vi "Main.vi"() -> ()   [LabVIEW 2018]
doc: "The myRIO Project template acquires acceleration data from the onboard accelerometer and displays the changes of acceleration values in a waveform chart."
uses:
  <vilib>/myRIO/Common/Instrument Driver Framework/myRIO v1.0/UART/vis/myRIO v1.0 Close UART.vi
  <vilib>/Utility/error.llb/Error Cluster From Error Code.vi
  <vilib>/myRIO/Common/Instrument Driver Framework/myRIO v1.0/PWM/vis/myRIO v1.0 Write PWM.vi
  <vilib>/myRIO/Common/Instrument Driver Framework/myRIO v1.0/DIO/vis/myRIO v1.0 Write DIO.vi
  <vilib>/myRIO/Common/Instrument Driver Framework/myRIO v1.0/AI/vis/myRIO v1.0 Read AI.vi
  <vilib>/myRIO/Common/Instrument Driver Framework/myRIO v1.0/DIO/vis/myRIO v1.0 Read DIO.vi
  <vilib>/myRIO/Common/Instrument Driver Framework/Utilities/vis/FPGA Ref Manager.vi
  <vilib>/myRIO/Common/Instrument Driver Framework/myRIO v1.0/myRIO v1.0 Reset FPGA.vi
  <vilib>/myRIO/Common/Instrument Driver Framework/myRIO v1.0/IRQ/vis/myRIO v1.0 IRQ Info FGV.vi
  <vilib>/myRIO/Common/Instrument Driver Framework/myRIO v1.0/IRQ/vis/myRIO v1.0 Timer IRQ Info FGV.vi
  <vilib>/myRIO/Common/Instrument Driver Framework/myRIO v1.0/IRQ/vis/myRIO v1.0 ISR Agent.vi
  <vilib>/myRIO/Instrument Drivers/Utilities/Utilities.lvlib
  <vilib>/myRIO/Instrument Drivers/Onboard IO/PWM/PWM.lvlib
  <vilib>/myRIO/Instrument Drivers/Onboard IO/AI/AI.lvlib
  <vilib>/myRIO/Instrument Drivers/Onboard IO/DIO/DIO.lvlib
panel:
  in  "ABORT STEPPER!!!!!":bool
  in  "Threshold Lower":dbl=2900.0
  in  "Threshold Upper":dbl=3200.0
  in  "Stepper frekvens":dbl=350.0
  out "ALL BOTTOM":bool
  out "ALL TOP":bool
  in  "Test bor (T = Amperestyring)":bool
  in  "DIR":bool
  in  "Endstops":bool
  in  "Manuel stepper?":bool
  in  "Enum":T1(ring)
  out "Batteri tilbage (%)":dbl
  out "Mean 200":dbl format="%0.2f"
  out "Duty Cycle":dbl
  in  "Styr manuelt?":bool=TRUE
  out "Waveform Chart":dbl(graph)
  out "Målt ampere":dbl
  in  "Bor - Frequency [Hz]":dbl=200.0
  in  "Bor - Duty Cycle":dbl=50.0
  out "error out":errorcluster
  in  "Stop":bool
  # "WIRING:\nBrun = GND\nOrange = PWM (A/DIO8)"
  # "STYRING AF SYSTEM!"
  # "100 = max\n50 = 0\n0 = -max"
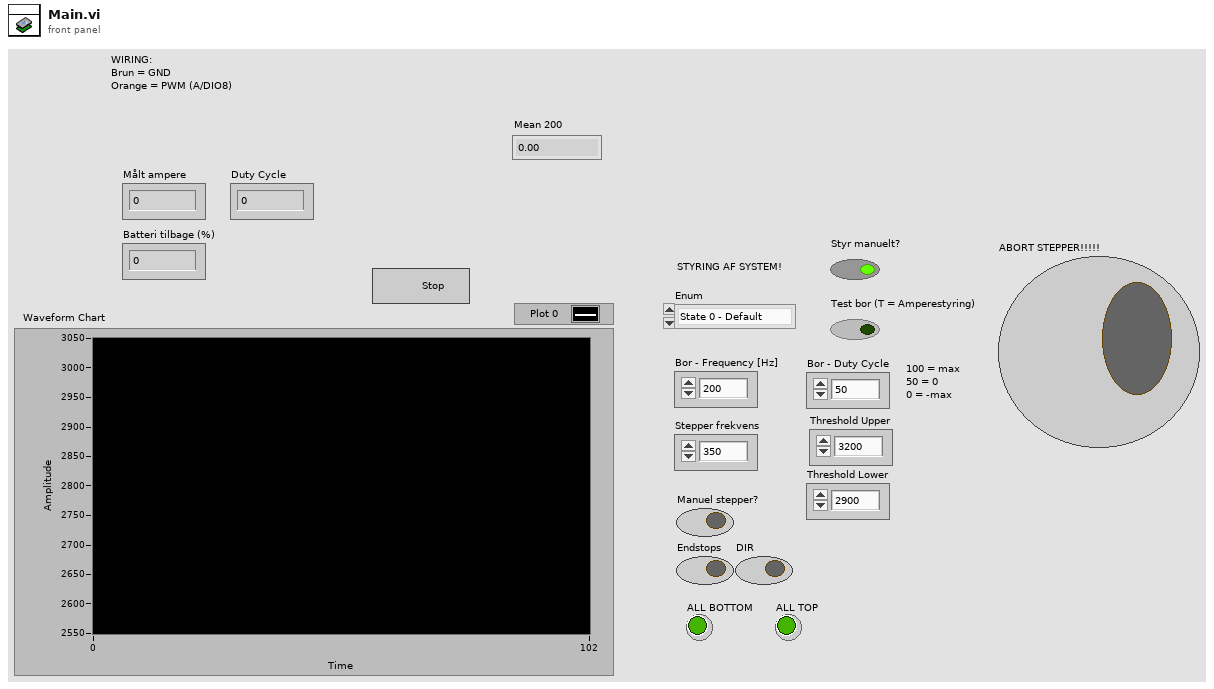
[diagram p1: front panel]
types:
  T1 = enum16{"State 0 - Default", "State 1 - Go down", "State 2 - Go up"}
  T2 = typedef "DIO.lvlib/DIO Reference.ctl" = cluster{"myRIO Reference":T3, "DIO Channels List":T7}
  T3 = typedef "myRIO Generic Hardware Reference.ctl" = cluster{"myRIO Model":T4, "myRIO Hardware Reference":T5}
  T4 = typedef "Hardware Version Enum.ctl" = enum16{"Unknown", "myRIO-1900", "myRIO-1950", "roboRIO", "NI ELVIS RIO CM", "ELVIS III"}
  T5 = typedef "myRIO v1.0 Reference.ctl" = cluster{"Generic FPGA Reference":T6, "Allow multiple opens":bool}
  T6 = typedef "Generic FPGA Reference.ctl" = refnum<k20>
  T7 = typedef "DIO Channels List.ctl" = T8[]
  T8 = typedef "DIO Channels Enum.ctl" = enum16{"Not Connected", "C/DIO0", "C/DIO1", "C/DIO2", "C/DIO3", "C/DIO4", "C/DIO5", "C/DIO6", "C/DIO7", "A/DIO0", "A/DIO1", "A/DIO2", "A/DIO3", "A/DIO4", "A/DIO5", "A/DIO6", "A/DIO7", "A/DIO8", "A/DIO9", "A/DIO10", "A/DIO11", "A/DIO12", "A/DIO13", "A/DIO14", "A/DIO15", "A/DIO16", "A/DIO17", "A/DIO18", "A/DIO19", "B/DIO0", "B/DIO1", "B/DIO2", "B/DIO3", "B/DIO4", "B/DIO5", "B/DIO6", "B/DIO7", "B/DIO8", "B/DIO9", "B/DIO10", "B/DIO11", "B/DIO12", "B/DIO13", "B/DIO14", "B/DIO15", "B/DIO16", "B/DIO17", "B/DIO18", "B/DIO19", "LED0", "LED1", "LED2", "LED3", "Button0", "DIO/DIO0", "DIO/DIO1", "DIO/DIO2", "DIO/DIO3", "DIO/DIO4", "DIO/DIO5", "DIO/DIO6", "DIO/DIO7", "DIO/DIO8", "DIO/DIO9", "SPI/CS0", "SPI/CS1", "SPI/CS2", "SPI/CS3", "LED RADIO (Green)", "LED RADIO (Red)", "LED COMM (Green)", "LED COMM (Red)", "LED MODE (Green)", "LED MODE (Red)"}
  T9 = typedef "PWM.lvlib/PWM Reference.ctl" = cluster{"myRIO Reference":T3, "PWM Channels Enum":T10, "PWM Configuration":T11}
  T10 = typedef "PWM Channels Enum.ctl" = enum16{"Not Connected", "C/PWM0", "C/PWM1", "A/PWM0", "A/PWM1", "A/PWM2", "A/PWM3", "A/PWM4", "A/PWM5", "A/PWM6", "A/PWM7", "A/PWM8", "A/PWM9", "A/PWM10", "A/PWM11", "A/PWM12", "A/PWM13", "A/PWM14", "A/PWM15", "A/PWM16", "A/PWM17", "A/PWM18", "A/PWM19", "B/PWM0", "B/PWM1", "B/PWM2", "B/PWM3", "B/PWM4", "B/PWM5", "B/PWM6", "B/PWM7", "B/PWM8", "B/PWM9", "B/PWM10", "B/PWM11", "B/PWM12", "B/PWM13", "B/PWM14", "B/PWM15", "B/PWM16", "B/PWM17", "B/PWM18", "B/PWM19", "PWM/PWM0", "PWM/PWM1", "PWM/PWM2", "PWM/PWM3", "PWM/PWM4", "PWM/PWM5", "PWM/PWM6", "PWM/PWM7", "PWM/PWM8", "PWM/PWM9"}
  T11 = typedef "PWM.lvlib/PWM Configuration.ctl" = cluster{"Frequency":dbl, "Duty Cycle":dbl}
  T12 = typedef "Accelerometer.lvlib/Accelerometer Reference.ctl" = cluster{"myRIO Reference":T3, "Accelerometer Channels List":T13, "LSB Weight":dbl}
  T13 = typedef "Accelerometer Channels List.ctl" = T14[]
  T14 = typedef "Accelerometer Channels Enum.ctl" = enum16{"Not Connected", "X-Axis", "Y-Axis", "Z-Axis"}
  T15 = typedef "AI.lvlib/AI Reference.ctl" = cluster{"myRIO Reference":T3, "AI Channels List":T16, "AI Scaling Constants List":T18}
  T16 = typedef "AI Channels List.ctl" = T17[]
  T17 = typedef "AI Channels Enum.ctl" = enum16{"Not Connected", "AudioIn/Left", "AudioIn/Right", "C/AI0", "C/AI1", "A/AI0", "A/AI1", "A/AI2", "A/AI3", "A/AI4", "A/AI5", "A/AI6", "A/AI7", "B/AI0", "B/AI1", "B/AI2", "B/AI3", "B/AI4", "B/AI5", "B/AI6", "B/AI7", "AI/AI0", "AI/AI1", "AI/AI2", "AI/AI3", "A/AI0 (DIFF)", "A/AI1 (DIFF)", "A/AI2 (DIFF)", "A/AI3 (DIFF)", "B/AI0 (DIFF)", "B/AI1 (DIFF)", "B/AI2 (DIFF)", "B/AI3 (DIFF)"}
  T18 = typedef "Analog Scaling Constants List.ctl" = T19[]
  T19 = typedef "Analog Scaling Constants.ctl" = cluster{"LSB Weight (Volts)":dbl, "Offset (Volts)":dbl, "Signed?":bool}
  T20 = typedef "SPI.lvlib/SPI Reference.ctl" = cluster{"myRIO Reference":T3, "SPI Channels Enum":T21, "SPI Configuration":T22}
  T21 = typedef "SPI Channels Enum.ctl" = enum16{"Not Connected", "A/SPI", "B/SPI", "SPI/SPI"}
  T22 = typedef "SPI.lvlib/SPI Configuration.ctl" = cluster{"Frequency [Hz]":dbl, "Clock Phase":T23, "Clock Polarity":T24, "Data Direction":T25, "Frame Length":T26}
  T23 = typedef "SPI Clock Phase.ctl" = enum8{"Leading", "Trailing"}
  T24 = typedef "SPI Clock Polarity.ctl" = enum8{"Low", "High"}
  T25 = typedef "SPI Data Direction.ctl" = enum8{"Most significant bit first", "Least significant bit first"}
  T26 = typedef "SPI Frame Length.ctl" = u8
  T27 = cluster{"B/DIO0 - Stepper Direction":T2, "B/DIO1 - Stepper1 Enable":T2, "B/DIO2 - Stepper2 Enable":T2, "B/DIO3 - Stepper3 Enable":T2, "B/DIO4 - Endstop Stepper1 Top":T2, "B/DIO11 - Endstop Stepper1 Bund":T2, "B/DIO12 - Endstop Stepper2 Top":T2, "B/DIO13 - Endstop Stepper2 Bund":T2, "B/DIO14 - Endstop Stepper3 Top":T2, "B/DIO15 - Endstop Stepper3 Bund":T2, "A/DIO0 - Cooler":T2, "A/DIO1 - Beacon drop (dio1)":T2, "A/DIO2 - Beacon drop (dio0)":T2, "A/DIO3 - QuickRelease (dio1)":T2, "A/DIO4 - QuickRelease (dio0)":T2, "A/DIO11 - LiDAR SPI CS":T2, "B/PWM0 - Stepper":T9, "B/PWM1 - Drill":T9, "A/PWM0 - Servo_Roll":T9, "A/PWM1 - Servo_Yaw":T9, "Acc. X-axis":T12, "Acc. Y-axis":T12, "B/AI0 - Drone Grounded F3":T15, "B/AI1 - Drone Drill Gear F4":T15, "B/AI2 - Beacon Drop F5":T15, "B/AI3 - Drone Drill Boost F6":T15, "A/AI0 - Drone Stepper F8":T15, "A/AI1 - Beacon Wiper":T15, "A/AI2 - QuickRelease Wiper":T15, "A/AI3 - Drill Current":T15, "A/SPI - LiDAR":T20, "B/UART - XBee":refnum<visa-resource-name>, "A/UART - A3 GPS":refnum<visa-resource-name>, "RIO Flashing LEDs":T2}
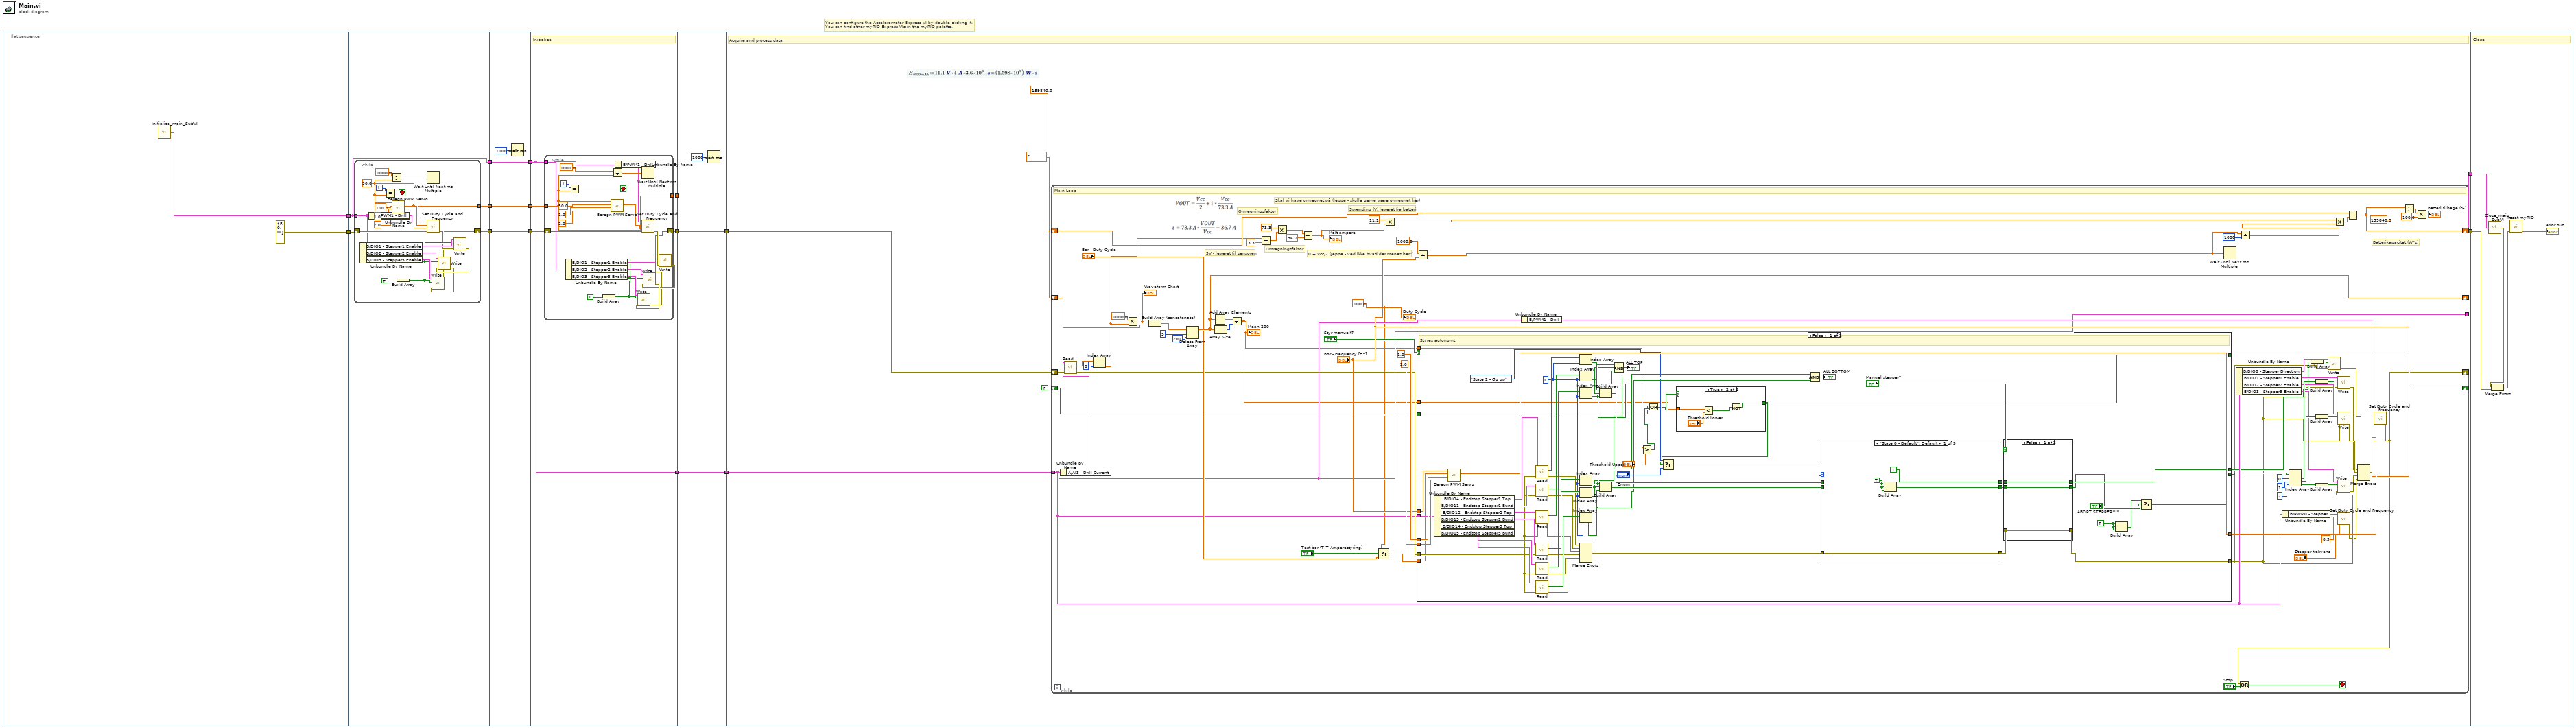
[diagram p0: block diagram]
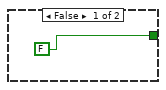
[diagram p2: hidden frame]
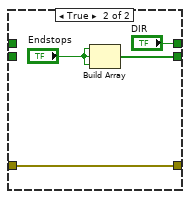
[diagram p3: hidden frame]
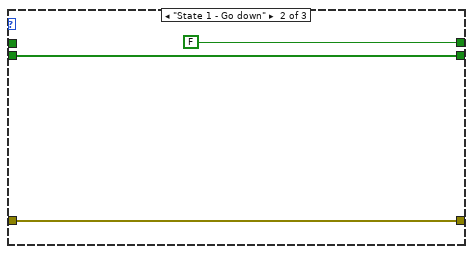
[diagram p4: hidden frame]
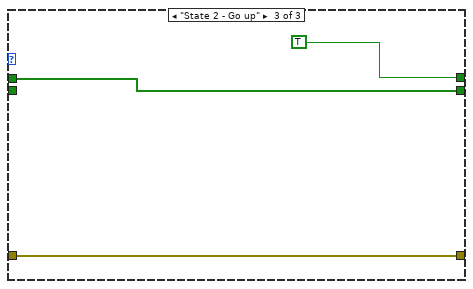
[diagram p5: hidden frame]
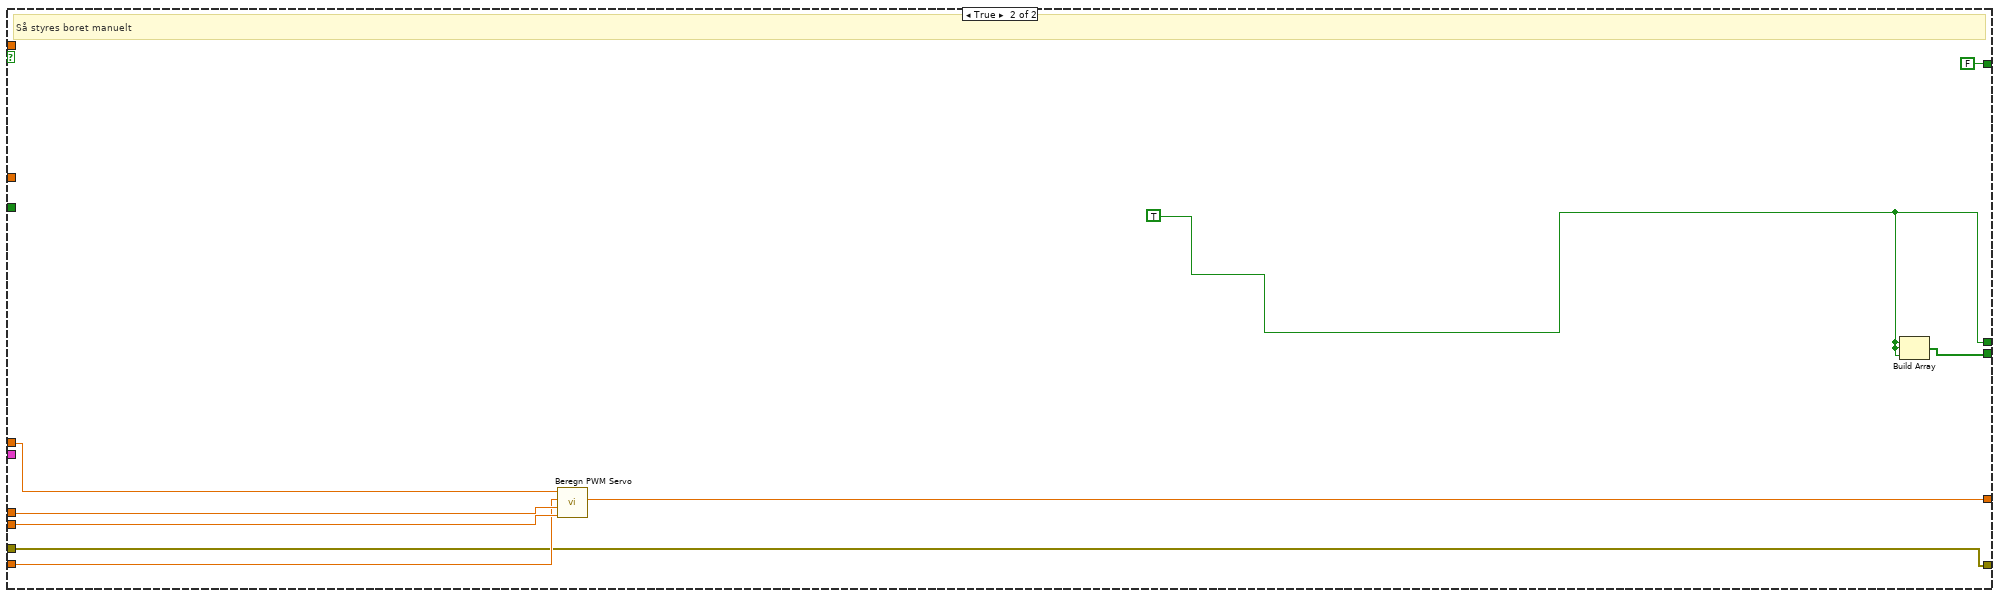
[diagram p6: hidden frame]
diagram:
  # "You can configure the Accelerometer Express VI by double-clicking it.\nYou can find other myRIO Express VIs in the myRIO palette."
  n1 = flat-sequence {
    tunnel: [w17] -> w8
    tunnel: [errorcluster {"status"=FALSE, "code"=0, "source"=""} ("error constant")] -> w2
    tunnel: [w21] -> w13
    tunnel: [w20] -> w11
    tunnel: w8 -> [w19]
    tunnel: [w19] -> w7
    tunnel: w2 -> [w18]
    tunnel: [w45] -> w14
    tunnel: w13 -> [w45]
    tunnel: [w44] -> w12
    tunnel: w11 -> [w44]
    tunnel: w7 -> [w43]
    tunnel: [w43] -> w6
    tunnel: w14 -> [w51]
    tunnel: w12 -> [w50]
    tunnel: [w48] -> w10
    tunnel: [w49] -> w9
    tunnel: w6 -> [w47]
    tunnel: [w47] -> w4
    tunnel: w10 -> [w73]
    tunnel: w9 -> [_]
    tunnel: [w74] -> w5
    tunnel: w4 -> [w74]
    tunnel: [w73] -> w3
    tunnel: [w82] -> w15
    tunnel: w5 -> [w79]
    tunnel: w3 -> [w78]
    tunnel: [w77] -> w1
    tunnel: w15 -> [w251]
    tunnel: w1 -> [w249]
    frame #0 {
      n2 = call "Initialize_main_SubVI.vi"() -> ("output cluster"=w17:T27)
    }
    frame #1 {
      n3 = while {
        tunnel: [w35] -> w21
        shift-right: [w22] -> w20
        shift-left: w18 -> [w38]
        tunnel: w19 -> [w31]
        i -> [w37]
        stop <- w33 stop-if-true
        w35 = 50.0 ("Frequency [Hz]")
        n4 = Unbundle By Name(w31) -> ("B/DIO1 - Stepper1 Enable"=w29:T2, "B/DIO2 - Stepper2 Enable"=w28:T2, "B/DIO3 - Stepper3 Enable"=w27:T2)
        n5 = Unbundle By Name(w31) -> ("B/PWM1 - Drill"=w32:T9)
        n6 = Equal?(x=w37, y=w35) -> (x = y?=w33:bool)
        n7 = Divide(x=1000.0, y=w35) -> (x/y=w36:dbl)
        n8 = call "Beregn PWM Servo.vi"("Max (ms puls bredde)"=2.0, "Min (ms puls bredde)"=1.0, "Duty Cycle"=100.0, "Frekvens"=w35) -> ("Output Dutycycle til PWM Servo"=w39:dbl)  [unwired: 7 in]
        n9 = Build Array(TRUE) -> (w26:bool[])
        n10 = Wait Until Next ms Multiple(millisecond multiple=w36) -> ()  [unwired: 1 out]
        n11 = call <vilib>:"Set Duty Cycle and Frequency.vi"("error in (no error)"=w38, "Frequency [Hz]"=w35, "Duty Cycle"=w39, "PWM Ref In"=w32) -> ("error out"=w25:errorcluster)  [unwired: 5 in, 1 out]
        n12 = call <vilib>:"Write.vi"("error in (no error)"=w25, "Values"=w26, "DIO Ref In"=w29) -> ("error out"=w24:errorcluster)  [unwired: 6 in, 1 out]
        n13 = call <vilib>:"Write.vi"("error in (no error)"=w24, "Values"=w26, "DIO Ref In"=w28) -> ("error out"=w23:errorcluster)  [unwired: 6 in, 1 out]
        n14 = call <vilib>:"Write.vi"("error in (no error)"=w23, "Values"=w26, "DIO Ref In"=w27) -> ("error out"=w22:errorcluster)  [unwired: 6 in, 1 out]
      }
    }
    frame #2 {
      n15 = Wait (ms)(milliseconds to wait=u32 1000) -> ()  [unwired: 1 out]
    }
    frame #3 {
      # "Initialize"
      n16 = while {
        tunnel: [w63] -> w49
        shift-right: [w54] -> w48
        shift-left: w50 -> [w68]
        tunnel: w51 -> [w63]
        tunnel: w47 -> [w56]
        i -> [w67]
        stop <- w64 stop-if-true
        n17 = Unbundle By Name(w56) -> ("B/DIO1 - Stepper1 Enable"=w53:T2, "B/DIO2 - Stepper2 Enable"=w58:T2, "B/DIO3 - Stepper3 Enable"=w59:T2)
        n18 = Equal?(x=w67, y=w63) -> (x = y?=w64:bool)
        n19 = Build Array(TRUE) -> (w52:bool[])
        n20 = call "Beregn PWM Servo.vi"("Max (ms puls bredde)"=2.0, "Min (ms puls bredde)"=1.0, "Duty Cycle"=50.0, "Frekvens"=w63) -> ("Output Dutycycle til PWM Servo"=w69:dbl)  [unwired: 7 in]
        n21 = Divide(x=1000.0, y=w63) -> (x/y=w66:dbl)
        n22 = Unbundle By Name(w56) -> ("B/PWM1 - Drill"=w62:T9)
        n23 = Wait Until Next ms Multiple(millisecond multiple=w66) -> ()  [unwired: 1 out]
        n24 = call <vilib>:"Set Duty Cycle and Frequency.vi"("error in (no error)"=w68, "Frequency [Hz]"=w63, "Duty Cycle"=w69, "PWM Ref In"=w62) -> ("error out"=w55:errorcluster)  [unwired: 5 in, 1 out]
        n25 = call <vilib>:"Write.vi"("error in (no error)"=w55, "Values"=w52, "DIO Ref In"=w53) -> ("error out"=w60:errorcluster)  [unwired: 6 in, 1 out]
        n26 = call <vilib>:"Write.vi"("error in (no error)"=w60, "Values"=w52, "DIO Ref In"=w58) -> ("error out"=w61:errorcluster)  [unwired: 6 in, 1 out]
        n27 = call <vilib>:"Write.vi"("error in (no error)"=w61, "Values"=w52, "DIO Ref In"=w59) -> ("error out"=w54:errorcluster)  [unwired: 6 in, 1 out]
      }
    }
    frame #4 {
      n28 = Wait (ms)(milliseconds to wait=u32 1000) -> ()  [unwired: 1 out]
    }
    frame #5 {
      # "Acquire and process data"
      n29 = while {
        shift-right: [w118] -> w82
        shift-left: w78 -> [w153]
        shift-right: [w143] -> _
        shift-left: dbl[] [] -> [w155]
        shift-right: [w128] -> _
        shift-left: 159840.0 -> [w129]
        tunnel: w79 -> [w115]
        tunnel: [w115] -> w77
        shift-right: [w86] -> _
        shift-left: FALSE ("t") -> [w85]
        stop <- w158 stop-if-true
        w83 = 100.0 ("upper limit")
        # "Batterikapacitet (W*s)"
        # "Spænding (V) leveret fra batteri"
        # "Omregningsfaktor"
        # "Omregningsfaktor"
        # "5V - leveret til sensoren"
        # "Skal vi have omregnet på (Jeppe - skulle gerne være omregnet her)"
        # "0 = Vcc/2 (Jeppe - ved ikke hvad der menes her?)"
        # "Main Loop"
        n30 = Unbundle By Name(w115) -> ("A/AI3 - Drill Current"=w121:T15)
        n31 = call <vilib>:"Read.vi"("error in (no error)"=w153, "AI Ref In"=w121) -> ("error out"=w119:errorcluster, "Values"=w152:dbl[])  [unwired: 7 in, 1 out]
        n32 = Index Array(array=w152, index=0) -> (element=w88:dbl)
        n33 = Multiply(x=1000.0, y=w88) -> (x*y=w141:dbl)
        "Waveform Chart" <- w141
        n34 = Build Array (concatenate)(w141, w155) -> (w146:dbl[])
        n35 = Delete From Array(array=w146, length=5, index=200) -> (array with subset deleted=w143:dbl[])  [unwired: 1 out]
        n36 = Add Array Elements(numeric array=w143) -> (sum=w145:dbl)
        n37 = Array Size(array=w143) -> (size(s)=w144:i32)
        n38 = Divide(x=w145, y=w144) -> (x/y=w84:dbl)
        "Mean 200" <- w84
        n39 = Divide(x=w88, y=3.3) -> (x/y=w139:dbl)
        n40 = Multiply(x=73.3, y=w139) -> (x*y=w137:dbl)
        n41 = Subtract(x=w137, y=36.7) -> (x-y=w134:dbl)
        "Målt ampere" <- w134
        n42 = Select(t=w83, s="Test bor (T = Amperestyring)", f="Bor - Duty Cycle") -> (s? t:f=w116:dbl)
        n43 = Multiply(x=11.1, y=w134) -> (x*y=w133:dbl)
        n44 = Divide(x=1000.0, y="Bor - Frequency [Hz]") -> (x/y=w87:dbl)
        n45 = case shown="False" "Styr manuelt?" {
          tunnel: 2.0 ("Max (ms puls bredde)") -> [w217 w248]
          tunnel: 1.0 ("Min (ms puls bredde)") -> [w215 w247]
          tunnel: [w214 w246] -> w151
          tunnel: "Bor - Frequency [Hz]" -> [w216 w245]
          tunnel: w115 -> [w195 _]
          tunnel: w119 -> [w194 w241]
          tunnel: w116 -> [w177 w244]
          tunnel: [w160 w242] -> w98
          tunnel: [w176 w241] -> w93
          tunnel: [w175 w243] -> w94
          tunnel: w84 -> [w171 _]
          tunnel: [w166 FALSE ("t")] -> w86
          tunnel: w85 -> [w169 _]
          tunnel: w84 -> [w167 _]
          frame False {
            w162 = TRUE
            w201 = 0 ("index")
            # "Styres autonomt"
            n46 = Unbundle By Name(w195) -> ("B/DIO4 - Endstop Stepper1 Top"=w213:T2, "B/DIO11 - Endstop Stepper1 Bund"=w212:T2, "B/DIO12 - Endstop Stepper2 Top"=w211:T2, "B/DIO13 - Endstop Stepper2 Bund"=w210:T2, "B/DIO14 - Endstop Stepper3 Top"=w209:T2, "B/DIO15 - Endstop Stepper3 Bund"=w208:T2)
            n47 = call "Beregn PWM Servo.vi"("Max (ms puls bredde)"=w217, "Min (ms puls bredde)"=w215, "Duty Cycle"=w177, "Frekvens"=w216) -> ("Output Dutycycle til PWM Servo"=w214:dbl)  [unwired: 7 in]
            n48 = call <vilib>:"Read.vi"("error in (no error)"=w194, "DIO Ref In"=w213) -> ("error out"=w193:errorcluster, "Values"=w202:bool[])  [unwired: 7 in, 1 out]
            n49 = call <vilib>:"Read.vi"("error in (no error)"=w194, "DIO Ref In"=w212) -> ("error out"=w192:errorcluster, "Values"=w203:bool[])  [unwired: 7 in, 1 out]
            n50 = call <vilib>:"Read.vi"("error in (no error)"=w194, "DIO Ref In"=w211) -> ("error out"=w191:errorcluster, "Values"=w204:bool[])  [unwired: 7 in, 1 out]
            n51 = call <vilib>:"Read.vi"("error in (no error)"=w194, "DIO Ref In"=w210) -> ("error out"=w190:errorcluster, "Values"=w205:bool[])  [unwired: 7 in, 1 out]
            n52 = call <vilib>:"Read.vi"("error in (no error)"=w194, "DIO Ref In"=w209) -> ("error out"=w189:errorcluster, "Values"=w206:bool[])  [unwired: 7 in, 1 out]
            n53 = call <vilib>:"Read.vi"("error in (no error)"=w194, "DIO Ref In"=w208) -> ("error out"=w188:errorcluster, "Values"=w207:bool[])  [unwired: 7 in, 1 out]
            n54 = Index Array(array=w202, index=w201) -> (element=w185:bool)
            n55 = Index Array(array=w204, index=w201) -> (element=w184:bool)
            n56 = Index Array(array=w206, index=w201) -> (element=w183:bool)
            n57 = Index Array(array=w203, index=w201) -> (element=w180:bool)
            n58 = Index Array(array=w205, index=w201) -> (element=w179:bool)
            n59 = Index Array(array=w207, index=w201) -> (element=w178:bool)
            n60 = Merge Errors(w193, w192, w191, w190, w189, w188) -> (w187:errorcluster)
            n61 = Build Array(w185, w184, w183) -> (w199:bool[])
            n62 = Build Array(w180, w179, w178) -> (w200:bool[])
            n63 = Compound Arithmetic op=AND(w185, w184, w183) -> (→"ALL TOP":bool)
            n64 = Greater?(x=w171, y="Threshold Upper") -> (0:w170:bool)
            n65 = Or(x=w169, y=w170) -> (x .or. y?=w168:bool)
            n66 = case shown="True" w168 {
              tunnel: [FALSE w219] -> w166
              tunnel: w167 -> [_ w221]
              frame False {
              }
              frame True {
                n67 = Less?(x=w221, y="Threshold Lower") -> (x < y?=w220:bool)
                n68 = Not(x=w220) -> (.not. x?=w219:bool)
              }
            }
            n69 = Select(t=T1."State 2 - Go up" ("Enum"), s=w166, f="Enum") -> (s? t:f=w165:T1)
            n70 = Compound Arithmetic op=AND(w180, w179, w178) -> (→"ALL BOTTOM":bool)
            n71 = case shown="\"State 0 - Default\", Default" w165 {
              tunnel: [w231 w236 w239] -> w197
              tunnel: w200 -> [_ w236 _]
              tunnel: w199 -> [_ _ w239]
              tunnel: [TRUE FALSE TRUE] -> w196
              tunnel: w187 -> [w230 w234 w237]
              tunnel: [w230 w234 w237] -> w186
              frame "State 0 - Default", Default {
                w232 = TRUE
                n72 = Build Array(w232, w232, w232) -> (w231:bool[])
              }
              frame "State 1 - Go down" {
              }
              frame "State 2 - Go up" {
              }
            }
            n73 = case shown="False" "Manuel stepper?" {
              tunnel: w197 -> [w225 _]
              tunnel: [w225 w229] -> w163
              tunnel: w196 -> [w224 _]
              tunnel: [w224 "DIR"] -> w175
              tunnel: w186 -> [w223 w226]
              tunnel: [w223 w226] -> w176
              frame False {
              }
              frame True {
                n74 = Build Array("Endstops", "Endstops", "Endstops") -> (w229:bool[])
              }
            }
            n75 = Build Array(w162, w162, w162) -> (w161:bool[])
            n76 = Select(t=w161, s="ABORT STEPPER!!!!!", f=w163) -> (s? t:f=w160:bool[])
          }
          frame True {
            w243 = TRUE ("DIR")
            # "Så styres boret manuelt"
            n77 = call "Beregn PWM Servo.vi"("Max (ms puls bredde)"=w248, "Min (ms puls bredde)"=w247, "Duty Cycle"=w244, "Frekvens"=w245) -> ("Output Dutycycle til PWM Servo"=w246:dbl)  [unwired: 7 in]
            n78 = Build Array(w243, w243, w243) -> (w242:bool[])
          }
        }
        n79 = Unbundle By Name(w115) -> ("B/PWM1 - Drill"=w120:T9)
        n80 = Wait Until Next ms Multiple(millisecond multiple=w87) -> ()  [unwired: 1 out]
        n81 = Unbundle By Name(w115) -> ("B/DIO0 - Stepper Direction"=w99:T2, "B/DIO1 - Stepper1 Enable"=w101:T2, "B/DIO2 - Stepper2 Enable"=w102:T2, "B/DIO3 - Stepper3 Enable"=w103:T2)
        n82 = Divide(x=w87, y=u32 1000) -> (x/y=w131:dbl)
        n83 = Unbundle By Name(w115) -> ("B/PWM0 - Stepper"=w114:T9)
        n84 = Index Array(array=w98, index #1=0 ("index"), index #2=1 ("index"), index #3=2 ("index")) -> (element #1=w104:bool, element #2=w106:bool, element #3=w108:bool)
        n85 = Build Array(w94) -> (w100:bool[])
        n86 = Build Array(w104) -> (w105:bool[])
        n87 = Build Array(w106) -> (w107:bool[])
        n88 = Build Array(w108) -> (w109:bool[])
        n89 = call <vilib>:"Write.vi"("error in (no error)"=w93, "Values"=w100, "DIO Ref In"=w99) -> ("error out"=w110:errorcluster)  [unwired: 6 in, 1 out]
        n90 = Multiply(x=w133, y=w131) -> (x*y=w130:dbl)
        n91 = call <vilib>:"Write.vi"("error in (no error)"=w93, "Values"=w105, "DIO Ref In"=w101) -> ("error out"=w111:errorcluster)  [unwired: 6 in, 1 out]
        n92 = call <vilib>:"Write.vi"("error in (no error)"=w93, "Values"=w107, "DIO Ref In"=w102) -> ("error out"=w112:errorcluster)  [unwired: 6 in, 1 out]
        n93 = call <vilib>:"Write.vi"("error in (no error)"=w93, "Values"=w109, "DIO Ref In"=w103) -> ("error out"=w90:errorcluster)  [unwired: 6 in, 1 out]
        n94 = call <vilib>:"Set Duty Cycle and Frequency.vi"("Frequency [Hz]"="Stepper frekvens", "Duty Cycle"=0.5, "PWM Ref In"=w114) -> ("error out"=w89:errorcluster)  [unwired: 6 in, 1 out]
        n95 = Subtract(x=w129, y=w130) -> (x-y=w128:dbl)
        n96 = Merge Errors(w110, w111, w112, w90, w89) -> (w92:errorcluster)
        n97 = call <vilib>:"Set Duty Cycle and Frequency.vi"("error in (no error)"=w92, "Frequency [Hz]"="Bor - Frequency [Hz]", "Duty Cycle"=w151, "PWM Ref In"=w120) -> ("error out"=w118:errorcluster)  [unwired: 5 in, 1 out]
        n98 = Or(x=w118, y="Stop") -> (x .or. y?=w158:bool)
        n99 = Divide(x=w128, y=159840.0) -> (x/y=w126:dbl)
        n100 = Multiply(x=w126, y=100.0) -> (x*y=→"Batteri tilbage (%)":dbl)
        "Duty Cycle" <- w83
      }
    }
    frame #6 {
      # "Close"
      n101 = call "Close_main_SubVI.vi"("output cluster"=w249) -> ("error constant"=w252:errorcluster)
      n102 = Merge Errors(w252, w251) -> (w250:errorcluster)
      n103 = call <vilib>:"Reset myRIO.vi"("error in (no error)"=w250) -> ("error out"=→"error out":errorcluster)  [unwired: 10 in]
    }
  }
